vi "transition_simple.vi"(4 "previous_state":T1, 6 "current_state":T1, 7 "transition_queue":refnum<queue>, 8 "error in (no error)":errorcluster, 9 "step":string, 10 "index in":i32, 11 "recipe_data in":variant) -> (0 "error out":errorcluster, 2 "index out":i32, 3 "recipe_data out":variant)   [LabVIEW 2015, in "example_01.lvlib"]
uses:
  example_01.lvlib
  <userlib>/antonio-alexander/lv-recipe-machine/public/_controls/automatic_state.ctl
  <userlib>/antonio-alexander/lv-recipe-machine/public/_controls/transition.ctl
  <userlib>/antonio-alexander/lv-recipe-machine/lv-recipe-machine.lvlib
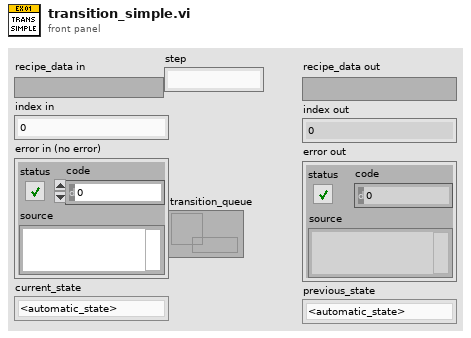
[diagram p1: front panel]
types:
  T1 = typedef "lv-recipe-machine.lvlib/automatic_state.ctl" = enum16{"<automatic_state>", "failed", "idle", "running", "paused", "stopped", "<null>"}
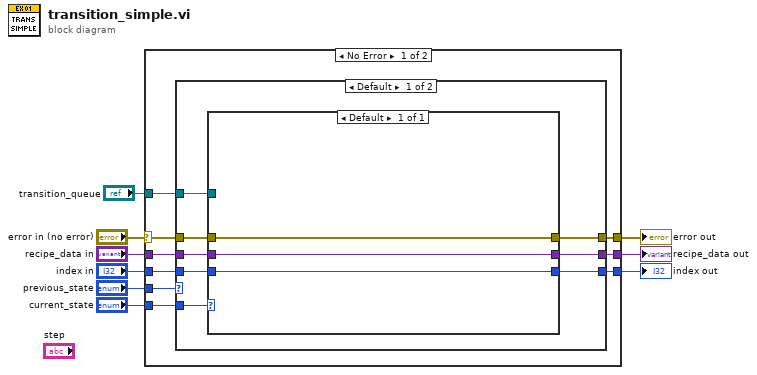
[diagram p0: block diagram]
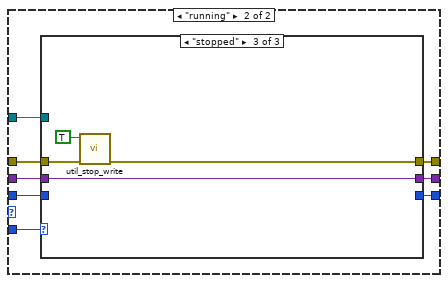
[diagram p2: hidden frame]
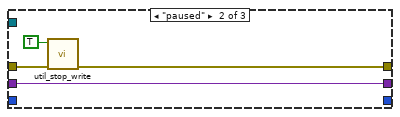
[diagram p4: hidden frame]
diagram:
  n1 = case shown="No Error" "error in (no error)" {
    selector: "error in (no error)" -> [w16 w51]
    tunnel: [w15 w51] -> w8
    tunnel: "recipe_data in" -> [w14 w50]
    tunnel: "index in" -> [w12 w49]
    tunnel: "current_state" -> [w17 _]
    tunnel: "previous_state" -> [w18 _]
    tunnel: [w13 w50] -> w3
    tunnel: [w11 w49] -> w2
    tunnel: "transition_queue" -> [w10 _]
    frame No Error {
      n2 = case shown="Default" w18 {
        tunnel: w17 -> [w26 w37]
        tunnel: w16 -> [w22 w33]
        tunnel: [w21 w32] -> w15
        tunnel: w14 -> [w24 w35]
        tunnel: [w23 w34] -> w13
        tunnel: w12 -> [w20 w31]
        tunnel: [w19 w30] -> w11
        tunnel: w10 -> [w25 w36]
        frame Default {
          n3 = case shown="Default" w26 {
            tunnel: w25 -> [_]
            tunnel: w24 -> [w29]
            tunnel: [w29] -> w23
            tunnel: w22 -> [w28]
            tunnel: [w28] -> w21
            tunnel: w20 -> [w27]
            tunnel: [w27] -> w19
            frame Default {
            }
          }
        }
        frame "running" {
          n4 = case shown="\"stopped\"" w37 {
            tunnel: w36 -> [_ _ _]
            tunnel: w35 -> [w40 w44 w48]
            tunnel: [w40 w44 w48] -> w34
            tunnel: w33 -> [w39 w42 w46]
            tunnel: [w39 w41 w45] -> w32
            tunnel: w31 -> [w38 _ _]
            tunnel: [w38 _ _] -> w30
            frame Default {
            }
            frame "paused" {
              n5 = call "util_stop_write.vi"("error in (no error)"=w42, "stop"=TRUE) -> ("error out"=w41:errorcluster)  [unwired: 9 in]
            }
            frame "stopped" {
              n6 = call "util_stop_write.vi"("error in (no error)"=w46, "stop"=TRUE) -> ("error out"=w45:errorcluster)  [unwired: 9 in]
            }
          }
        }
      }
    }
    frame Error {
    }
  }
  "error out" <- w8
  "recipe_data out" <- w3
  "index out" <- w2
